vi "new Bus Monitor.vi"(8 "error in":errorcluster, 9 "statistics (F)":bool, 11 "name":string) -> (0 "error out":errorcluster, 3 "busMonitor out":refnum<k24>)   [LabVIEW 2020, in "Ballard_1553_Hardware_ni.lvlib"]
uses:
  Ballard_1553_Hardware_ni.lvlib
  C:/Users/Administrator/Desktop/GIT/Ballard-MIL-STD-1553-Custom-Device/Source/System Explorer/SubVIs/Parse XML Ballard/1.2/BTIXML_SerDes.dll
  Ballard-MIL-STD-1553-Custom-Device/Source/System Explorer/SubVIs/Parse XML Ballard/1.2/BTIXML_SerDes.dll
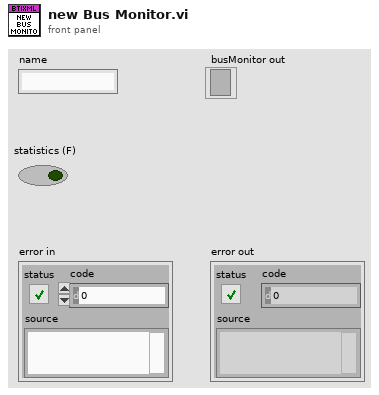
[diagram p1: front panel]
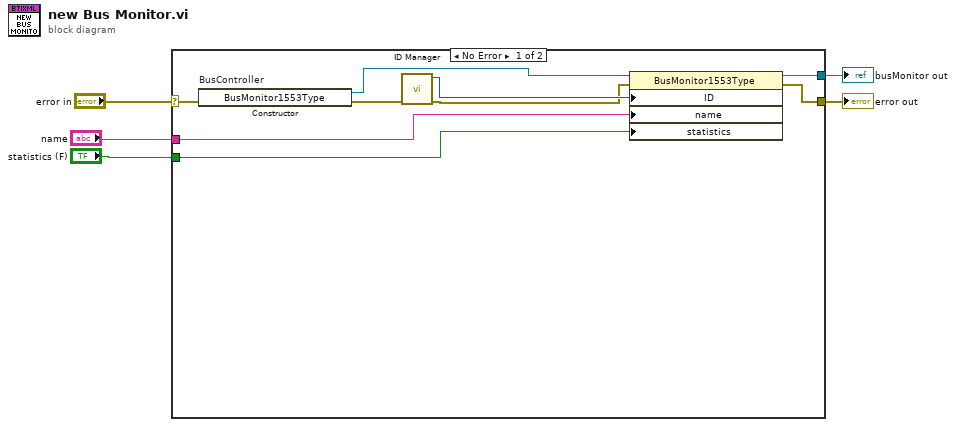
[diagram p0: block diagram]
diagram:
  n1 = case shown="No Error" "error in" {
    selector: "error in" -> [w14 w15]
    tunnel: [w13 w15] -> w4
    tunnel: [w12 _] -> w1
    tunnel: "statistics (F)" -> [w7 _]
    tunnel: "name" -> [w6 _]
    frame No Error {
      n2 = constructor on="BusController" class="BusMonitor1553Type"(error in=w14) -> (reference out=w11:refnum<k24>, error out=w10:errorcluster)  [unwired: 2 in, 1 out]
      n3 = call "ID Manager.vi"("error in"=w10) -> ("error out"=w8:errorcluster, "ID out"=w9:i32)  [unwired: 9 in]
      n4 = property class="BusMonitor1553Type"(reference=w11, error in=w8, "ID"=w9, "name"=w6, "statistics"=w7) -> (reference out=w12:refnum<k24>, error out=w13:errorcluster)
    }
    frame Error {
    }
  }
  "error out" <- w4
  "busMonitor out" <- w1
